vi "HMS_IPConfig_Verify_DHCP_Enabled.vi"(5 "error in (no error)":errorcluster) -> (14 "standard error":string, 15 "standard output":string, 16 "IP Reset":bool, 17 "DHCP Enabled":bool, 18 "PASS?":bool, 19 "error out":errorcluster)   [LabVIEW 2016]
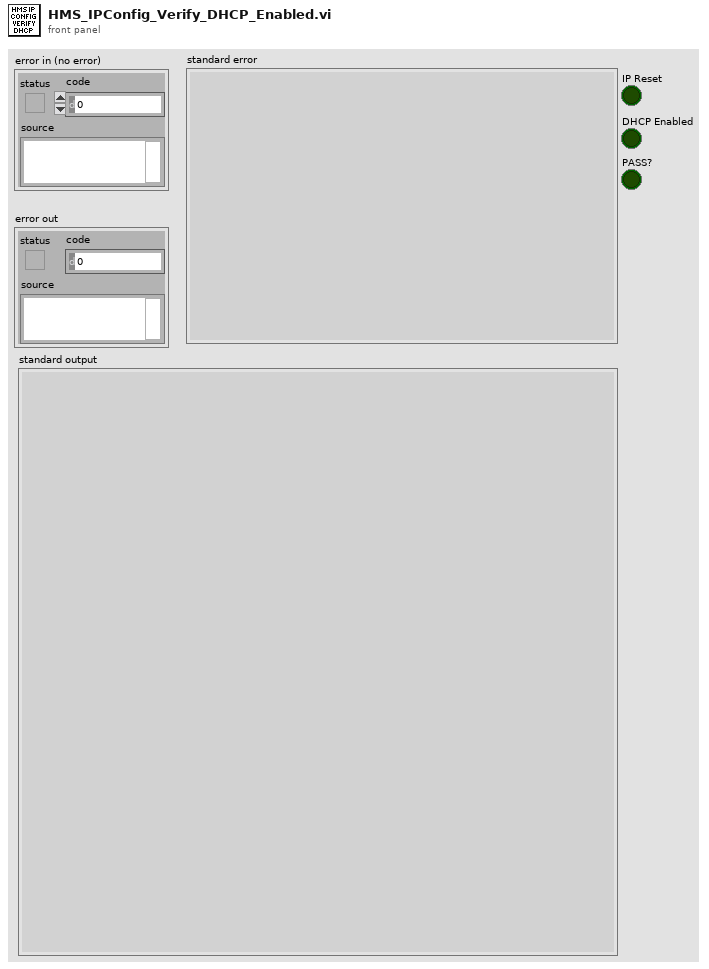
[diagram p1: front panel]
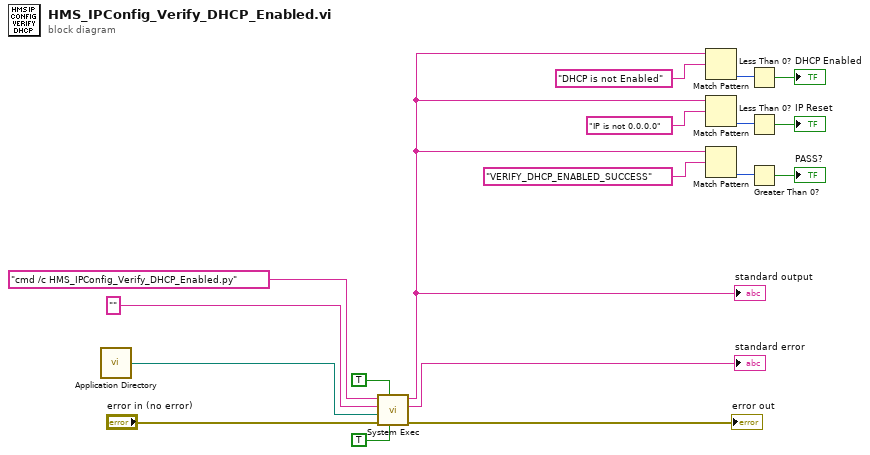
[diagram p0: block diagram]
diagram:
  n1 = call <vilib>:"Application Directory.vi"() -> ("Application Directory"=w1:path)
  n2 = call <vilib>:"System Exec.vi"("run minimized? (F)"=TRUE, "wait until completion? (T)"=TRUE ("run minimized? (F)"), "error in (no error)"="error in (no error)", "working directory"=w1, "standard input"="", "command line"="cmd /c HMS_IPConfig_Verify_DHCP_Enabled.py" ("name or relative path")) -> ("error out"=→"error out":errorcluster, "standard error"=→"standard error":string, "standard output"=w2:string)  [unwired: 2 in, 1 out]
  "standard output" <- w2
  n3 = Match Pattern(string=w2, regular expression="DHCP is not Enabled") -> (offset past match=w4:i32)  [unwired: 1 in, 3 out]
  n4 = Match Pattern(string=w2, regular expression="IP is not 0.0.0.0") -> (offset past match=w7:i32)  [unwired: 1 in, 3 out]
  n5 = Match Pattern(string=w2, regular expression="VERIFY_DHCP_ENABLED_SUCCESS") -> (offset past match=w10:i32)  [unwired: 1 in, 3 out]
  n6 = Less Than 0?(x=w4) -> (x < 0?=→"DHCP Enabled":bool)
  n7 = Less Than 0?(x=w7) -> (x < 0?=→"IP Reset":bool)
  n8 = Greater Than 0?(x=w10) -> (x > 0?=→"PASS?":bool)
